vi "write_attributes.vi"(8 "error in (no error)":errorcluster caption="entrée d'erreur (pas d'erreur)", 10 "attributes":T1, 11 "ARDRegression en entrée":refnum<class "ARDRegression.lvclass">) -> (0 "error out":errorcluster caption="sortie d'erreur", 3 "ARDRegression en sortie":refnum<class "ARDRegression.lvclass">)   [LabVIEW 2020, in "ARDRegression.lvclass"]
uses:
  ARDRegression.lvclass
  Controls/ardregressor_attributes.ctl
  ARDRegression.lvclass/ARDRegression.ctl
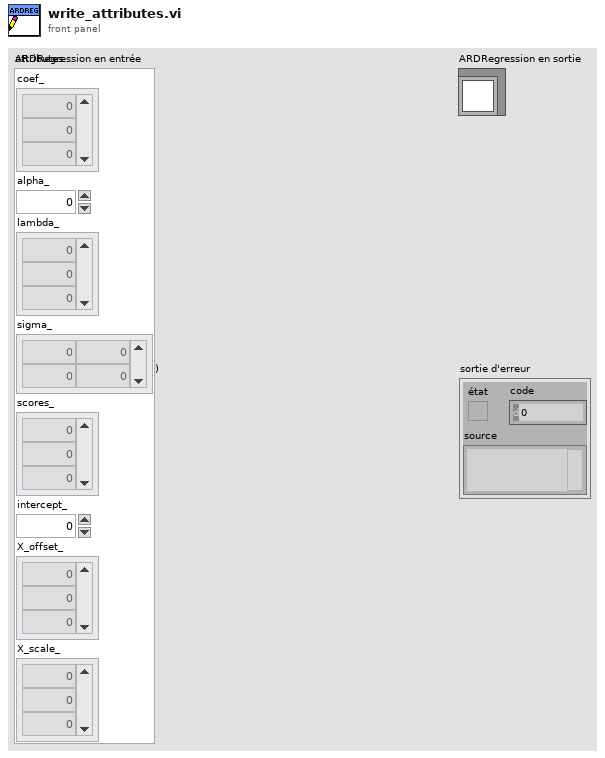
[diagram p1: front panel]
types:
  T1 = typedef "ardregressor_attributes.ctl" = cluster{"coef_":dbl[], "alpha_":dbl, "lambda_":dbl[], "sigma_":dbl[][], "scores_":dbl[], "intercept_":dbl, "X_offset_":dbl[], "X_scale_":dbl[]}
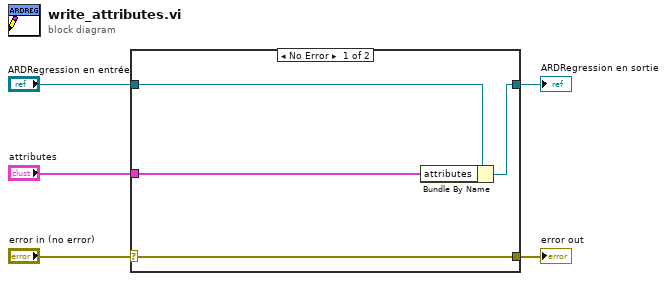
[diagram p0: block diagram]
diagram:
  n1 = case shown="No Error" "error in (no error)" {
    selector: "error in (no error)" -> [w9 w10]
    tunnel: [w9 w10] -> w4
    tunnel: [w7 w11] -> w2
    tunnel: "ARDRegression en entrée" -> [w8 w11]
    tunnel: "attributes" -> [w6 _]
    frame No Error {
      n2 = Bundle By Name(cluster=w8, "attributes"=w6) -> (w7:refnum<class "ARDRegression.lvclass">)
    }
    frame Error {
    }
  }
  "error out" <- w4
  "ARDRegression en sortie" <- w2
